vi "ConvertStartbit.vi"() -> ()   [LabVIEW 2021]
panel:
  out "Intel\nMSB":u16
  in  "Länge":u16=14
  out "Motorola\nMSB":u16=28
  out "Motorola\nLSB":u16
  in  "Intel Startbit\nLSB":u16
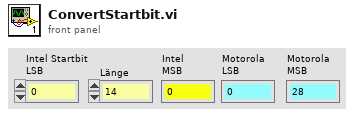
[diagram p1: front panel]
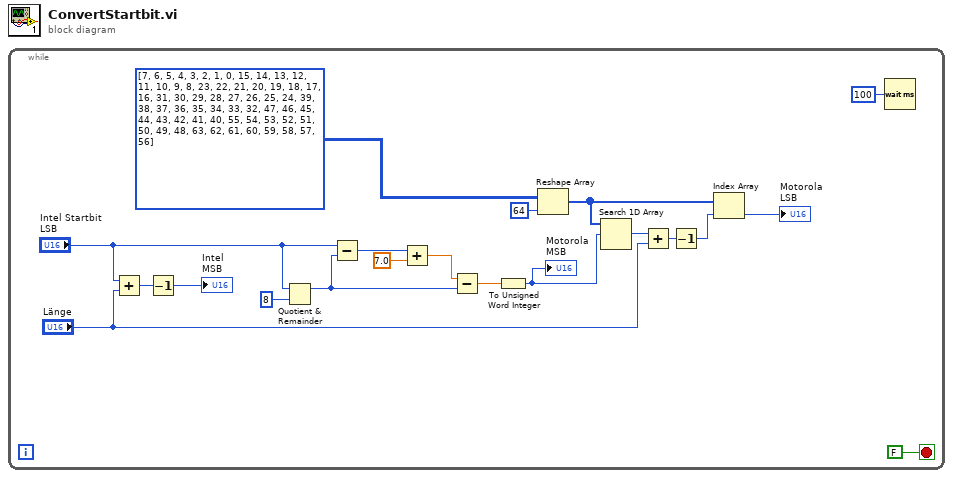
[diagram p0: block diagram]
diagram:
  n1 = while {
    stop <- FALSE stop-if-true
    n2 = Add(x="Intel Startbit\nLSB", y="Länge") -> (x+y=w3:u16)
    n3 = Decrement(x=w3) -> (x-1=→"Intel\nMSB":u16)
    n4 = Quotient & Remainder(x="Intel Startbit\nLSB", y=u16 8) -> (x-y*floor(x/y)=w13:u16)  [unwired: 1 out]
    n5 = Subtract(x="Intel Startbit\nLSB", y=w13) -> (x-y=w17:u16)
    n6 = Add(x=w17, y=7.0) -> (x+y=w15:dbl)
    n7 = Subtract(x=w15, y=w13) -> (x-y=w7:dbl)
    n8 = To Unsigned Word Integer(number=w7) -> (unsigned 16bit integer=w6:u16)
    "Motorola\nMSB" <- w6
    n9 = Reshape Array(u16[][] [[7, 6, 5, 4, 3, 2, 1, 0], [15, 14, 13, 12, 11, 10, 9, 8], [23, 22, 21, 20, 19, 18, 17, 16], [31, 30, 29, 28, 27, 26, 25, 24], [39, 38, 37, 36, 35, 34, 33, 32], [47, 46, 45, 44, 43, 42, 41, 40], [55, 54, 53, 52, 51, 50, 49, 48], [63, 62, 61, 60, 59, 58, 57, 56]] ("Array"), 64 ("Dimension")) -> (w8:u16[])
    n10 = Search 1D Array(1D array=w8, element=w6) -> (index of element=w12:i32)  [unwired: 1 in]
    n11 = Add(x=w12, y="Länge") -> (x+y=w11:i32)
    n12 = Decrement(x=w11) -> (x-1=w10:i32)
    n13 = Index Array(array=w8, index=w10) -> (element=→"Motorola\nLSB":u16)
    n14 = Wait (ms)(milliseconds to wait=u32 100 ("Zu wartende ms")) -> ()  [unwired: 1 out]
  }
